vi "asio_out_in.vi"(6 "error play 4":errorcluster, 7 "信号时长":dbl caption="等待时间（秒）" format="%#_6p", 8 "Format":cluster{"Rate":i32, "Bits":i32, "Channels":u32}={"Rate"=44100, "Bits"=32, "Channels"=2}, 9 "card #":u32, 10 "data_length":i32, 11 "output data":i32[][](array[numeric])) -> (2 "error play 2":errorcluster, 3 "error play 3":errorcluster, 4 "MIC_Data_IN":dbl[][](array[numeric]))   [LabVIEW 2018]
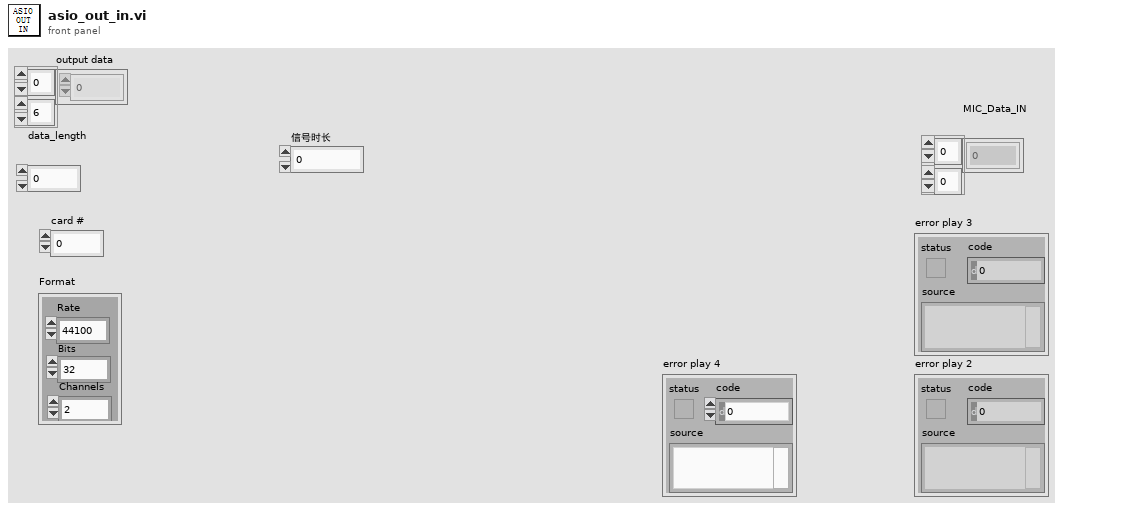
[diagram p1: front panel]
types:
  T1 = cluster{"# buffers":i32, "Buffer size":i32, "unit (ms)":enum16{"time (ms)", "Samples"}}
  T2 = typedef "SoundHandle.ctl" = cluster{"DeviceID":u16, "Samples/buf":u32, "Sampl rate":u32, "Bits/sample":u16, "Channels":u8, "Opened":bool}
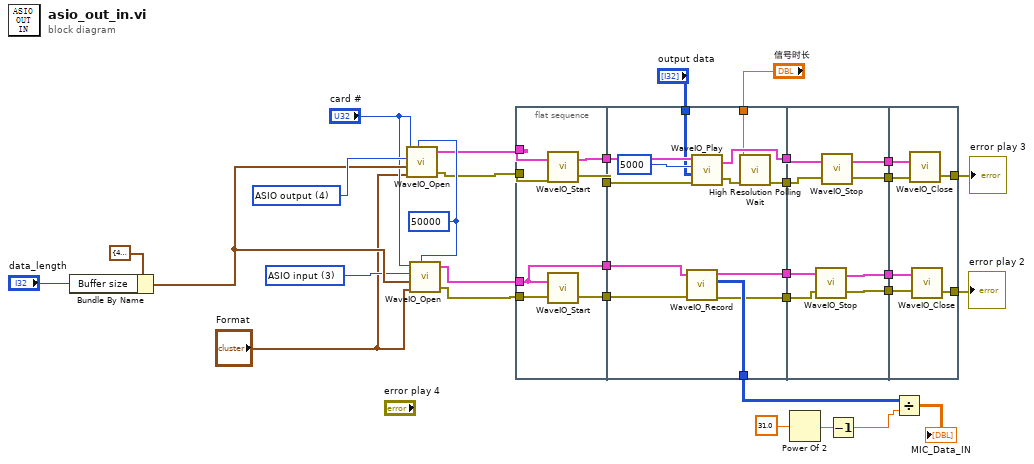
[diagram p0: block diagram]
diagram:
  w21 = u16 4 items=["Record", "Play", "Loopback", "ASIO input", "ASIO output", "Record (WASAPI)", "Play (WASAPI)", "Record Combi", "Play Combi"] ("device type (Record)")
  w14 = u16 3 items=["Record", "Play", "Loopback", "ASIO input", "ASIO output", "Record (WASAPI)", "Play (WASAPI)", "Record Combi", "Play Combi"] ("device type (Record)")
  w17 = 50000 ("Watchdog timeout (msec) (default=OFF)")
  n1 = Bundle By Name(cluster=T1 {"# buffers"=4, "Buffer size"=88200, "unit (ms)"=enum."Samples"} ("Buffer"), "Buffer size"="data_length") -> (w19:T1)
  n2 = call "WaveIO_Open.vi"("idev"="card #", "Watchdog timeout (msec) (default=OFF)"=w17, "device type (Record)"=w21, "Buffer Config"=w19, "Format (44kHz, 16Bit, stereo)"="Format") -> ("Sound Handle Out"=w11:T2, "error out"=w12:errorcluster)  [unwired: 2 in]
  n3 = call "WaveIO_Open.vi"("idev"="card #", "Watchdog timeout (msec) (default=OFF)"=w17, "device type (Record)"=w14, "Buffer Config"=w19, "Format (44kHz, 16Bit, stereo)"="Format") -> ("Sound Handle Out"=w13:T2, "error out"=w1:errorcluster)  [unwired: 2 in]
  n4 = flat-sequence {
    tunnel: [w37] -> w33
    tunnel: [w38] -> w32
    tunnel: w12 -> [w40]
    tunnel: w11 -> [w39]
    tunnel: w1 -> [w36]
    tunnel: w13 -> [w35]
    tunnel: [w35] -> w31
    tunnel: [w34] -> w30
    tunnel: [w48] -> w29
    tunnel: [w49] -> w28
    tunnel: w33 -> [w53]
    tunnel: w32 -> [w52]
    tunnel: w31 -> [w47]
    tunnel: w30 -> [w46]
    tunnel: [w45] -> w20
    tunnel: [w44] -> w27
    tunnel: [w43] -> w26
    tunnel: "信号时长" -> [w42]
    tunnel: "output data" -> [w41]
    tunnel: w29 -> [w57]
    tunnel: w28 -> [w56]
    tunnel: w27 -> [w61]
    tunnel: w26 -> [w60]
    tunnel: [w59] -> w25
    tunnel: [w58] -> w24
    tunnel: [w55] -> w23
    tunnel: [w54] -> w22
    tunnel: w25 -> [w67]
    tunnel: w24 -> [w66]
    tunnel: [w65] -> w10
    tunnel: w23 -> [w64]
    tunnel: w22 -> [w63]
    tunnel: [w62] -> w16
    frame #0 {
      n5 = call "WaveIO_Start.vi"("error in (no error)"=w40, "Handle"=w39) -> ("error out"=w38:errorcluster, "Handle Out"=w37:T2)
      n6 = call "WaveIO_Start.vi"("error in (no error)"=w36, "Handle"=w35) -> ("error out"=w34:errorcluster)  [unwired: 1 out]
    }
    frame #1 {
      n7 = call "WaveIO_Record.vi"("Handle"=w47, "error in (no error)"=w46) -> ("Handle Out"=w44:T2, "Data"=w45:i32[][], "error out"=w43:errorcluster)  [unwired: 1 in, 2 out]
      n8 = call "WaveIO_Play.vi"("error in (no error)"=w52, "data"=w41, "timeout (automatic)"=5000, "Handle"=w53) -> ("error out"=w50:errorcluster, "Handle Out"=w48:T2)
      n9 = call <vilib>:"High Resolution Polling Wait.vi"("error in (no error)"=w50, "seconds to wait"=w42) -> ("error out"=w49:errorcluster)  [unwired: 9 in]
    }
    frame #2 {
      n10 = call "WaveIO_Stop.vi"("error in (no error)"=w60, "Handle"=w61) -> ("error out"=w58:errorcluster, "Handle Out"=w59:T2)
      n11 = call "WaveIO_Stop.vi"("error in (no error)"=w56, "Handle"=w57) -> ("error out"=w54:errorcluster, "Handle Out"=w55:T2)
    }
    frame #3 {
      n12 = call "WaveIO_Close.vi"("error in (no error)"=w63, "Handle"=w64) -> ("error out"=w62:errorcluster)  [unwired: 1 out]
      n13 = call "WaveIO_Close.vi"("error in (no error)"=w66, "Handle"=w67) -> ("error out"=w65:errorcluster)  [unwired: 1 out]
    }
  }
  n14 = Power Of 2(x=31.0) -> (2^x=w8:dbl)
  n15 = Decrement(x=w8) -> (x-1=w7:dbl)
  n16 = Divide(x=w20, y=w7) -> (x/y=→"MIC_Data_IN":dbl[][])
  "error play 2" <- w10
  "error play 3" <- w16
